vi "LimelightAutoTracking.vi"() -> ()   [LabVIEW 2018]
uses:
  <vilib>/addons/control/pid/NI_PID_pid.lvlib
  <vilib>/addons/control/pid/pid.llb/PID (DBL).vi
panel:
  in  "horizontalAvgSize":i32
  out "PID Output":dbl(graph)
  in  "PID gains":T1={"proportional gain (Kc)"=1.0, "integral time (Ti, min)"=0.01, "derivative time (Td, min)"=0.0} {"derivative time (Td, min)" format="%.3f"; "integral time (Ti, min)" format="%.3f"; "proportional gain (Kc)" format="%.3f"}
  out "Camera X":T2(graph)
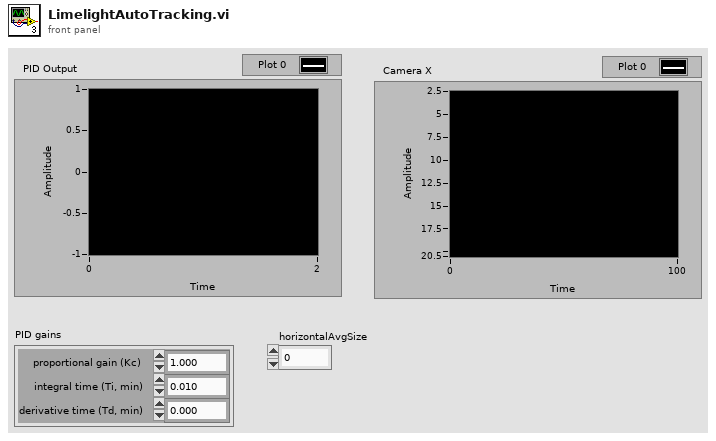
[diagram p1: front panel]
types:
  T1 = cluster{"proportional gain (Kc)":dbl, "integral time (Ti, min)":dbl, "derivative time (Td, min)":dbl}
  T2 = cluster{"offsetAngle H":dbl, "setpoint":dbl, dbl}
  T3 = cluster{"Horizontal Offset":dbl, "Vertical Offset":dbl, "Skew":dbl, "Area":dbl, "Valid?":bool}
  T4 = cluster{"Horizontal Offset":dbl, "setpoint":dbl, "Double":dbl}
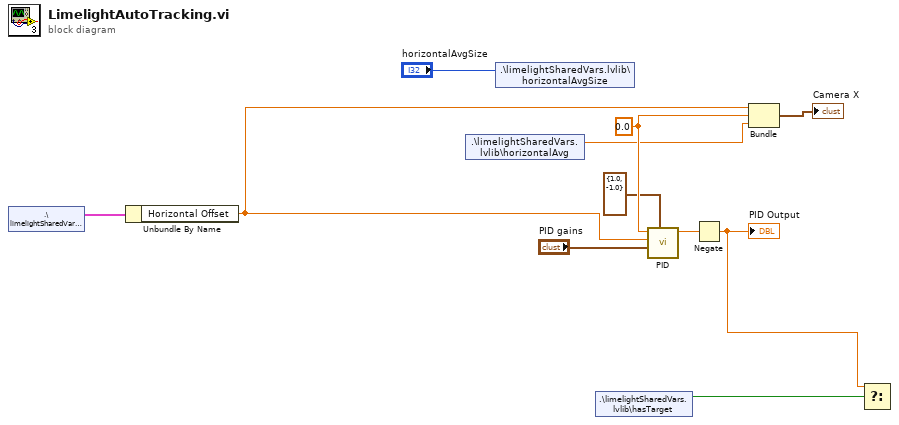
[diagram p0: block diagram]
diagram:
  w9 = 0.0 ("setpoint")
  n1 = shared-variable ".\\limelightSharedVars.lvlib\\target"() -> (w4:T3)  [unwired: 1 in, 1 out]
  n2 = Unbundle By Name(w4) -> ("Horizontal Offset"=w3:dbl)
  n3 = shared-variable ".\\limelightSharedVars.lvlib\\horizontalAvg"() -> (w5:dbl)  [unwired: 1 in, 1 out]
  n4 = shared-variable ".\\limelightSharedVars.lvlib\\horizontalAvgSize"("horizontalAvgSize") -> ()  [unwired: 1 in, 1 out]
  n5 = shared-variable ".\\limelightSharedVars.lvlib\\hasTarget"() -> (w11:bool)  [unwired: 1 in, 1 out]
  n6 = call-poly <vilib>:"PID.vi"("output range"=cluster{"output high":dbl, "output low":dbl} {"output high"=1.0, "output low"=-1.0}, "PID gains"="PID gains", "process variable"=w3, "setpoint"=w9) -> ("output"=w10:dbl)  [unwired: 6 in, 1 out]
  n7 = Negate(x=w10) -> (-x=w1:dbl)
  "PID Output" <- w1
  n8 = Bundle("Horizontal Offset"=w3, "setpoint"=w9, "Double"=w5) -> (→"Camera X":T4)  [unwired: 1 in]
  n9 = Select(t=w1, s=w11) -> ()  [unwired: 1 in, 1 out]
